vi "AddText2Image.vi"(8 "error in (no error)":errorcluster, 10 "TextOnImage":T1={"Status"="Stopped", "Experiment Name"="Experimt", "Current Temp (C)"="23.3", "Mag"="x50", "Set Point (C)"="23.3", "Cooling Rate (C/min)"="x50"}, 11 "Input Image":T2) -> (0 "error out":errorcluster, 3 "Output Image":T2)   [LabVIEW 2013]
doc: "Use this template to build a VI to use as a subVI."
uses:
  <vilib>/vision/Image Controls.llb/IMAQ Image.ctl
  TextOnImage.ctl
  <vilib>/vision/NI_Vision_Development_Module.lvlib
panel:
  out "Reference Image":T2(plugin-control)
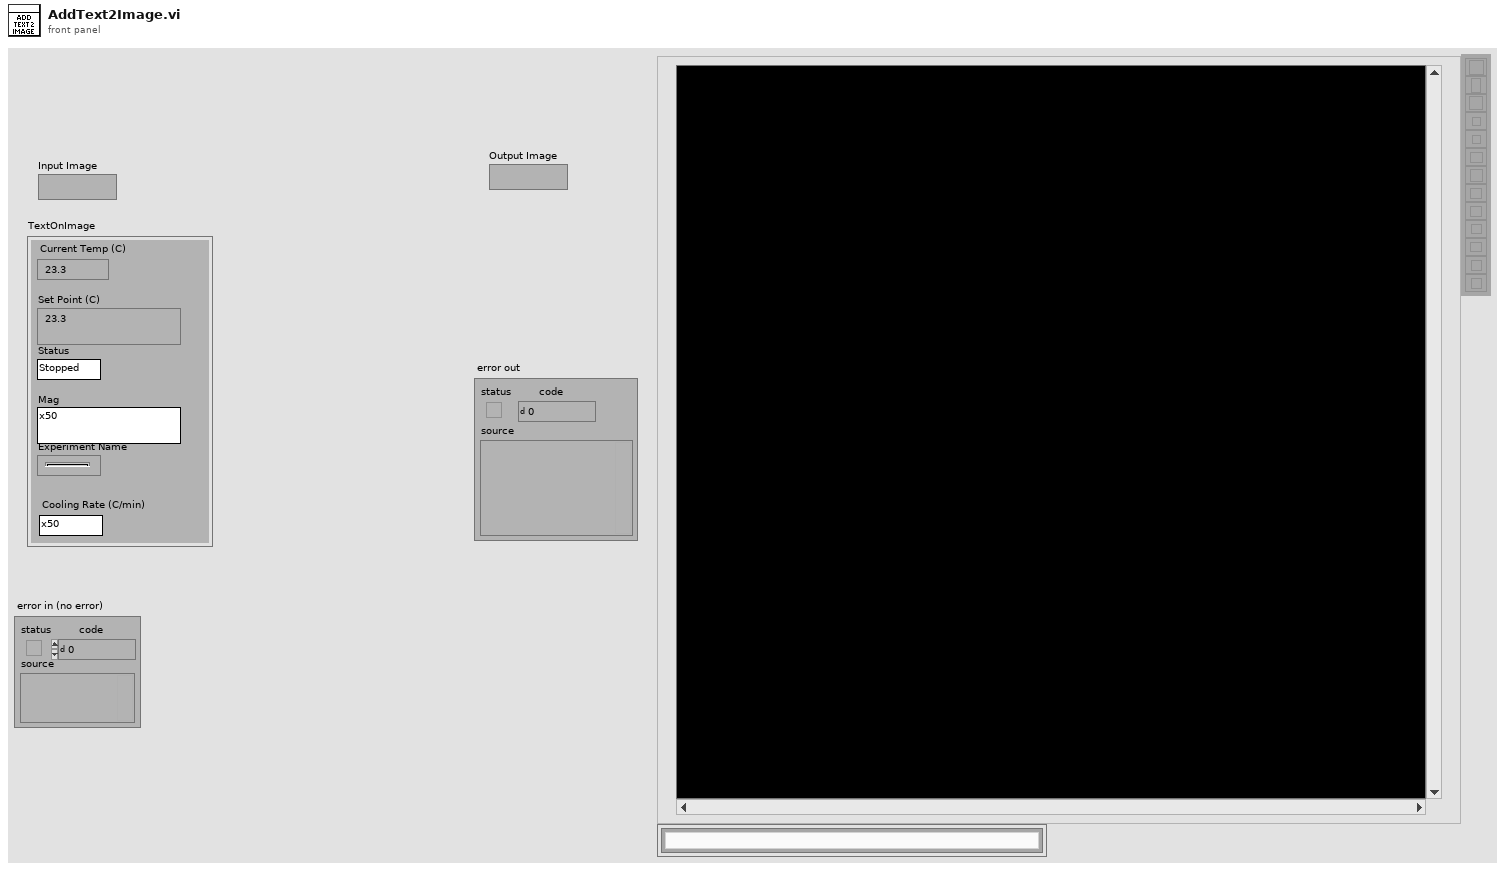
[diagram p1: front panel]
types:
  T1 = typedef "TextOnImage.ctl" = cluster{"Status":string, "Experiment Name":string, "Current Temp (C)":string, "Mag":string, "Set Point (C)":string, "Cooling Rate (C/min)":string}
  T2 = typedef "IMAQ Image.ctl" = refnum<image>
  T3 = cluster{"Desired Font (Application)":enum16{"User-specified Font", "Application Font", "System Font", "Dialog Font"}, "[User-specified Font]":cluster{"Font Name":string, "Size":i16, "Strikeout?":bool, "Italic?":bool, "Underline?":bool, "Outline?":bool, "Shadow?":bool, "Bold?":bool, "Rotation Angle":dbl}, "Horizontal Alignment":i16, "Vertical Alignment":i16}
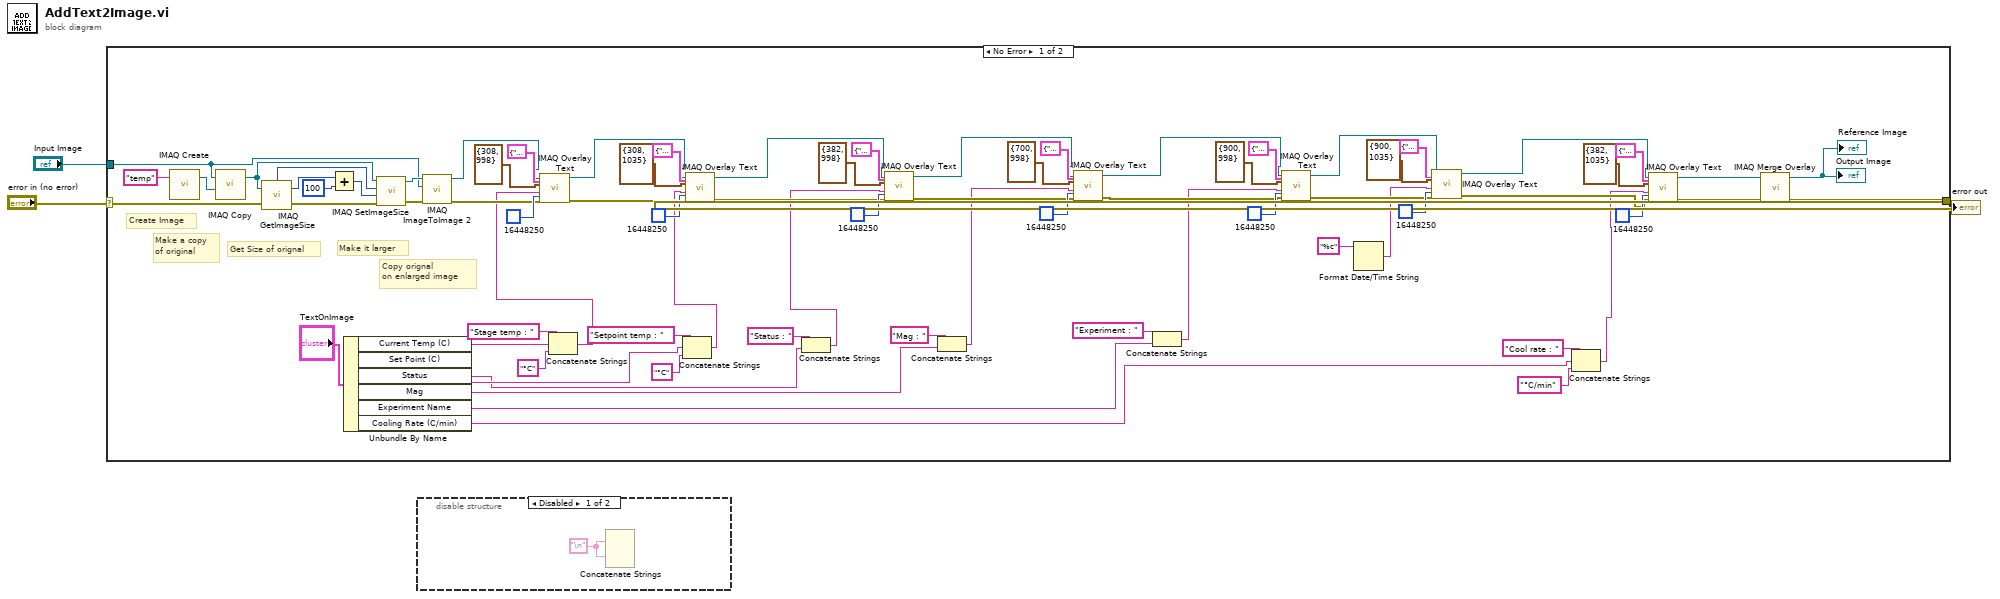
[diagram p0: block diagram]
diagram:
  n1 = case shown="No Error" "error in (no error)" {
    selector: "error in (no error)" -> [w78 w79]
    tunnel: [w65 w79] -> w2
    tunnel: "Input Image" -> [w67 _]
    frame No Error {
      # "Copy orignal\non enlarged image"
      # "Make it larger"
      # "Get Size of orignal"
      # "Make a copy\nof original"
      # "Create Image"
      n2 = call "IMAQ Create"("Image Name"="temp") -> ("New Image"=w69:T2)  [unwired: 4 in, 1 out]
      n3 = call "IMAQ Copy"("Image Dst"=w69, "Image Src"=w67) -> ("Image Dst Out"=w68:T2)  [unwired: 4 in, 1 out]
      n4 = call "IMAQ GetImageSize"("Image"=w68, "error in (no error)"=w78) -> ("Y Resolution"=w75:i32, "X Resolution"=w77:i32, "error out"=w76:errorcluster)  [unwired: 2 in]
      n5 = Add(x=w75, y=100) -> (x+y=w73:i32)
      n6 = Unbundle By Name("TextOnImage") -> ("Current Temp (C)"=w57:string, "Set Point (C)"=w47:string, "Status"=w39:string, "Mag"=w31:string, "Experiment Name"=w23:string, "Cooling Rate (C/min)"=w5:string)
      n7 = call "IMAQ SetImageSize"("error in (no error)"=w76, "Y Resolution"=w73, "X Resolution"=w77, "Image"=w68) -> ("error out"=w70:errorcluster, "Image Out"=w71:T2)  [unwired: 1 in]
      n8 = call "IMAQ ImageToImage 2"("error in (no error)"=w70, "Image Src (Small)"=w67, "Image Src (Large)"=w71) -> ("error out"=w60:errorcluster, "Image Dst Out"=w59:T2)  [unwired: 7 in]
      n9 = Concatenate Strings("Stage temp : " ("string"), w57, "°C" ("string")) -> (w56:string)
      n10 = call "IMAQ Overlay Text"("Text Color (black)"=u32 16448250, "Font, Size & Style"=T3 {"Desired Font (Application)"=enum."User-specified Font", "[User-specified Font]"={"Font Name"="", "Size"=32, "Strikeout?"=FALSE, "Italic?"=FALSE, "Underline?"=FALSE, "Outline?"=FALSE, "Shadow?"=FALSE, "Bold?"=TRUE, "Rotation Angle"=0.0}, "Horizontal Alignment"=2, "Vertical Alignment"=2}, "error in (no error)"=w60, "String"=w56, "Origin"=cluster{"X":i32, "Y":i32} {"X"=308, "Y"=998}, "Image"=w59) -> ("error out"=w50:errorcluster, "Image Out"=w51:T2)  [unwired: 4 in]
      n11 = Concatenate Strings("Setpoint temp : " ("string"), w47, "°C" ("string")) -> (w46:string)
      n12 = call "IMAQ Overlay Text"("Text Color (black)"=u32 16448250, "Font, Size & Style"=T3 {"Desired Font (Application)"=enum."User-specified Font", "[User-specified Font]"={"Font Name"="", "Size"=32, "Strikeout?"=FALSE, "Italic?"=FALSE, "Underline?"=FALSE, "Outline?"=FALSE, "Shadow?"=FALSE, "Bold?"=TRUE, "Rotation Angle"=0.0}, "Horizontal Alignment"=2, "Vertical Alignment"=2}, "error in (no error)"=w50, "String"=w46, "Origin"=cluster{"X":i32, "Y":i32} {"X"=308, "Y"=1035}, "Image"=w51) -> ("error out"=w42:errorcluster, "Image Out"=w41:T2)  [unwired: 4 in]
      n13 = Concatenate Strings("Status : " ("string"), w39) -> (w38:string)
      n14 = call "IMAQ Overlay Text"("Text Color (black)"=u32 16448250, "Font, Size & Style"=T3 {"Desired Font (Application)"=enum."User-specified Font", "[User-specified Font]"={"Font Name"="", "Size"=32, "Strikeout?"=FALSE, "Italic?"=FALSE, "Underline?"=FALSE, "Outline?"=FALSE, "Shadow?"=FALSE, "Bold?"=TRUE, "Rotation Angle"=0.0}, "Horizontal Alignment"=0, "Vertical Alignment"=2}, "error in (no error)"=w42, "String"=w38, "Origin"=cluster{"X":i32, "Y":i32} {"X"=382, "Y"=998}, "Image"=w41) -> ("error out"=w33:errorcluster, "Image Out"=w34:T2)  [unwired: 4 in]
      n15 = Concatenate Strings("Mag : " ("string"), w31) -> (w30:string)
      n16 = call "IMAQ Overlay Text"("Text Color (black)"=u32 16448250, "Font, Size & Style"=T3 {"Desired Font (Application)"=enum."User-specified Font", "[User-specified Font]"={"Font Name"="", "Size"=32, "Strikeout?"=FALSE, "Italic?"=FALSE, "Underline?"=FALSE, "Outline?"=FALSE, "Shadow?"=FALSE, "Bold?"=TRUE, "Rotation Angle"=0.0}, "Horizontal Alignment"=0, "Vertical Alignment"=2}, "error in (no error)"=w33, "String"=w30, "Origin"=cluster{"X":i32, "Y":i32} {"X"=700, "Y"=998}, "Image"=w34) -> ("error out"=w25:errorcluster, "Image Out"=w26:T2)  [unwired: 4 in]
      n17 = Concatenate Strings("Experiment : " ("string"), w23) -> (w22:string)
      n18 = call "IMAQ Overlay Text"("Text Color (black)"=u32 16448250, "Font, Size & Style"=T3 {"Desired Font (Application)"=enum."User-specified Font", "[User-specified Font]"={"Font Name"="", "Size"=32, "Strikeout?"=FALSE, "Italic?"=FALSE, "Underline?"=FALSE, "Outline?"=FALSE, "Shadow?"=FALSE, "Bold?"=TRUE, "Rotation Angle"=0.0}, "Horizontal Alignment"=0, "Vertical Alignment"=2}, "error in (no error)"=w25, "String"=w22, "Origin"=cluster{"X":i32, "Y":i32} {"X"=900, "Y"=998}, "Image"=w26) -> ("error out"=w17:errorcluster, "Image Out"=w18:T2)  [unwired: 4 in]
      n19 = Format Date/Time String(time format string (%c)="%c") -> (date/time string=w15:string)  [unwired: 2 in]
      n20 = call "IMAQ Overlay Text"("Text Color (black)"=u32 16448250, "Font, Size & Style"=T3 {"Desired Font (Application)"=enum."User-specified Font", "[User-specified Font]"={"Font Name"="", "Size"=32, "Strikeout?"=FALSE, "Italic?"=FALSE, "Underline?"=FALSE, "Outline?"=FALSE, "Shadow?"=FALSE, "Bold?"=TRUE, "Rotation Angle"=0.0}, "Horizontal Alignment"=0, "Vertical Alignment"=2}, "error in (no error)"=w17, "String"=w15, "Origin"=cluster{"X":i32, "Y":i32} {"X"=900, "Y"=1035}, "Image"=w18) -> ("error out"=w10:errorcluster, "Image Out"=w11:T2)  [unwired: 4 in]
      n21 = Concatenate Strings("Cool rate : " ("string"), w5, "°C/min" ("string")) -> (w4:string)
      n22 = call "IMAQ Overlay Text"("Text Color (black)"=u32 16448250, "Font, Size & Style"=T3 {"Desired Font (Application)"=enum."User-specified Font", "[User-specified Font]"={"Font Name"="", "Size"=32, "Strikeout?"=FALSE, "Italic?"=FALSE, "Underline?"=FALSE, "Outline?"=FALSE, "Shadow?"=FALSE, "Bold?"=TRUE, "Rotation Angle"=0.0}, "Horizontal Alignment"=0, "Vertical Alignment"=2}, "error in (no error)"=w10, "String"=w4, "Origin"=cluster{"X":i32, "Y":i32} {"X"=382, "Y"=1035}, "Image"=w11) -> ("error out"=w8:errorcluster, "Image Out"=w9:T2)  [unwired: 4 in]
      n23 = call "IMAQ Merge Overlay"("error in (no error)"=w8, "Image Src"=w9) -> ("error out"=w65:errorcluster, "Image Dst Out"=→"Output Image" →"Reference Image":T2)  [unwired: 8 in]
    }
    frame Error {
    }
  }
  "error out" <- w2
  n24 = disable-structure shown="Disabled" {
    frame Disabled {
      w80 = "\n"
      n25 = Concatenate Strings(w80, w80) -> ()  [unwired: 3 in, 1 out]
    }
    frame Enabled {
    }
  }
